vi "Execute.vi"(8 "error in (no error)":errorcluster, 10 "Context in":refnum<class "Context.lvclass">, 11 "Move Steps Command in":refnum<class "Move Steps Command.lvclass">) -> (0 "error out":errorcluster, 2 "Context out":refnum<class "Context.lvclass">, 3 "Move Steps Command out":refnum<class "Move Steps Command.lvclass">)   [LabVIEW 2016, in "Move Steps Command.lvclass"]
uses:
  Move Steps Command.lvclass
  Context/Context.lvclass
  Move Steps Command.lvclass/Move Steps Command.ctl
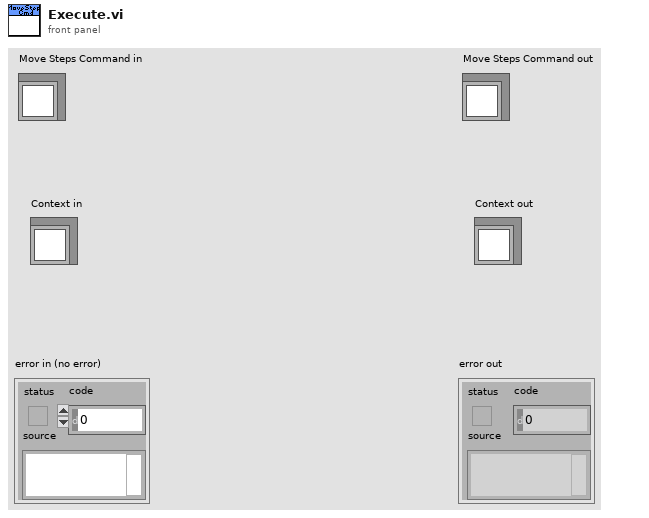
[diagram p1: front panel]
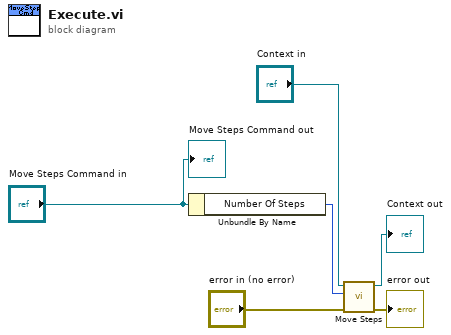
[diagram p0: block diagram]
diagram:
  n1 = Unbundle By Name("Move Steps Command in") -> ("Number Of Steps"=w2:i32)
  n2 = call "Move Steps.vi"("error in (no error)"="error in (no error)", "Number Of Steps"=w2, "Context in"="Context in") -> ("error out"=→"error out":errorcluster, "Context out"=→"Context out":refnum<class "Context.lvclass">)  [unwired: 7 in]
  "Move Steps Command out" <- "Move Steps Command in"
